vi "SH_Clustering.vi"(0 "Array of Shapelets in":cluster{dbl[][]}[](array[cluster]), 1 "NumberOfShapelets":i32, 3 "error in":errorcluster) -> (7 "Array of Shapelets out":cluster{dbl[][]}[](array[cluster]), 8 "Deleted shapelets":i32[](array[numeric]), 10 "error out":errorcluster)   [LabVIEW 2016, in "Shapelets Search (Brute Force).lvlib"]
uses:
  <vilib>/Analysis/Matrix/Datatypes/RealMatrix.ctl
  Shapelets Search (Brute Force).lvlib
  <vilib>/Analysis/Matrix/NI_Matrix.lvlib
panel:
  out "Real Matrix":T1
  # "This VI is a part of BCI Design library, http://www.ru-bci.org \nCopyright © 2020, Sotnikov Peter, All rights reserved. License: GNU GPLv3"
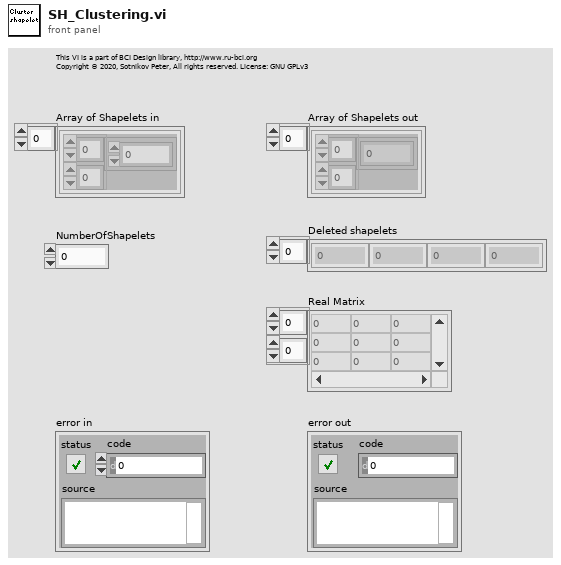
[diagram p1: front panel]
types:
  T1 = typedef "NI_Matrix.lvlib/RealMatrix.ctl" = dbl[][]
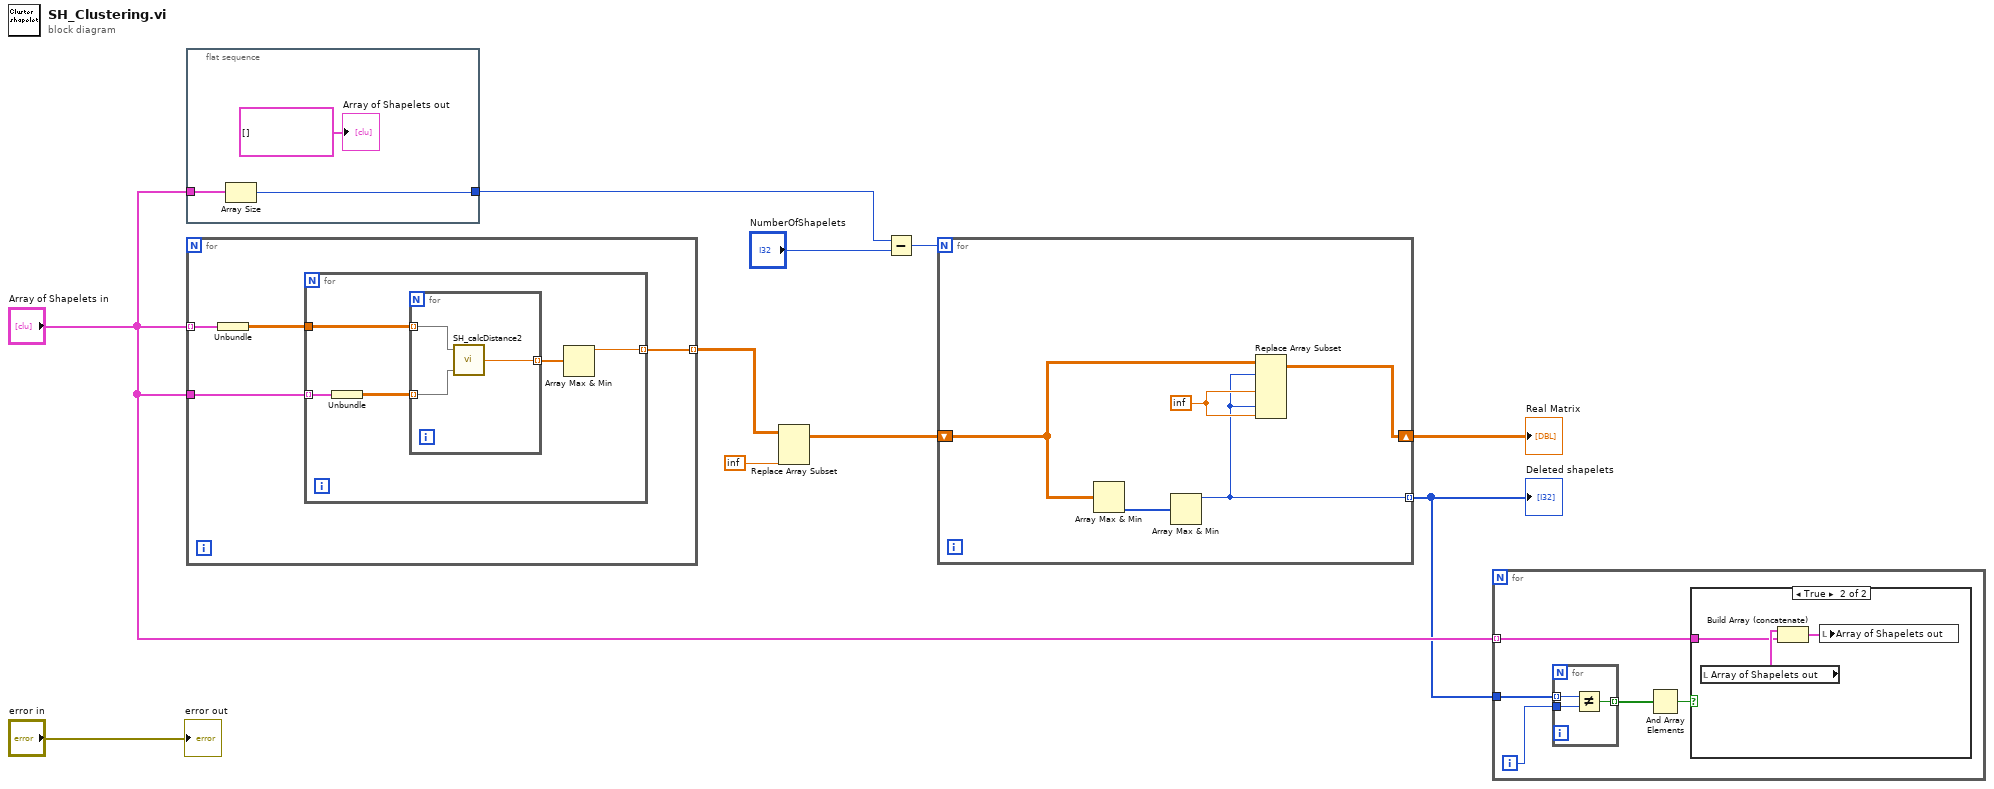
[diagram p0: block diagram]
diagram:
  n1 = flat-sequence {
    tunnel: [w11] -> w4
    tunnel: "Array of Shapelets in" -> [w13]
    frame #0 {
      n2 = Array Size(array=w13) -> (size(s)=w11:i32)
      "Array of Shapelets out" <- cluster{dbl[][]}[] [] ("Array of Shapelets out")
    }
  }
  n3 = for {
    tunnel: "Array of Shapelets in" -> [w17] mode=indexing
    tunnel: "Array of Shapelets in" -> [w16]
    tunnel: [w14] -> w6 mode=indexing
    n4 = Unbundle(w17) -> (w15:dbl[][])
    n5 = for {
      tunnel: w16 -> [w22] mode=indexing
      tunnel: w15 -> [w21]
      tunnel: [w18] -> w14 mode=indexing
      n6 = Unbundle(w22) -> (w20:dbl[][])
      n7 = for {
        tunnel: w21 -> [w25] mode=indexing
        tunnel: w20 -> [w24] mode=indexing
        tunnel: [w23] -> w19 mode=indexing
        n8 = call "SH_calcDistance2.vi"("Shapelet 2"=w24, "Shapelet 1"=w25) -> ("Distance out"=w23:dbl)  [unwired: 1 in]
      }
      n9 = Array Max & Min(array=w19) -> (max value=w18:dbl)  [unwired: 3 out]
    }
  }
  n10 = Replace Array Subset(array=w6, new element=inf) -> (w8:T1)  [unwired: 2 in]
  n11 = Subtract(x=w4, y="NumberOfShapelets") -> (x-y=w5:i32)
  n12 = for {
    N: w5 -> [_]
    shift-right: [w28] -> w7
    shift-left: w8 -> [w30]
    tunnel: [w26] -> w1 mode=indexing
    w29 = inf
    n13 = Array Max & Min(array=w30) -> (min index (indices)=w27:i32[])  [unwired: 3 out]
    n14 = Array Max & Min(array=w27) -> (max value=w26:i32)  [unwired: 3 out]
    n15 = Replace Array Subset(array=w30, new element #1=w29, index (row) #1=w26, new element #2=w29, index (col) #2=w26) -> (w28:T1)  [unwired: 2 in]
  }
  "Real Matrix" <- w7
  "Deleted shapelets" <- w1
  n16 = for {
    tunnel: w1 -> [w34]
    tunnel: "Array of Shapelets in" -> [w31] mode=indexing
    i -> [w35]
    n17 = for {
      tunnel: w35 -> [w40]
      tunnel: w34 -> [w41] mode=indexing
      tunnel: [w39] -> w33 mode=indexing
      n18 = Not Equal?(x=w41, y=w40) -> (x != y?=w39:bool)
    }
    n19 = And Array Elements(Boolean array=w33) -> (logical AND=w32:bool)
    n20 = case shown="True" w32 {
      tunnel: w31 -> [_ w36]
      frame False {
      }
      frame True {
        n21 = local read "Array of Shapelets out"() -> (w37:cluster{dbl[][]}[])
        n22 = Build Array (concatenate)(w37, w36) -> (w38:cluster{dbl[][]}[])
        n23 = local write "Array of Shapelets out"(w38) -> ()
      }
    }
  }
  "error out" <- "error in"
